vi "Init Any Page.vi"(8 "error in (no error)":errorcluster, 11 "VI in":refnum<vi>) -> (1 "Page Ctrl #N Ref":refnum<vi>, 2 "Page Ctrl #1 Ref":refnum<vi>)   [LabVIEW 2016]
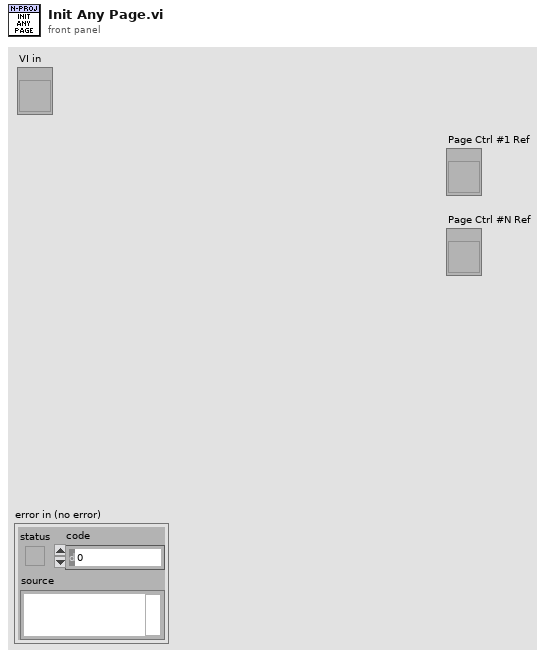
[diagram p1: front panel]
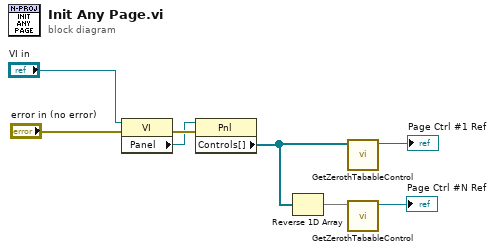
[diagram p0: block diagram]
diagram:
  n1 = property class="VI"(reference="VI in", error in="error in (no error)") -> (error out=w4:errorcluster, "Panel"=w3:refnum<vi>)  [unwired: 1 out]
  n2 = property class="Pnl"(reference=w3, error in=w4) -> ("Controls[]"=w6:refnum<vi>[])  [unwired: 2 out]
  n3 = Reverse 1D Array(array=w6) -> (reversed array=w7:refnum<vi>[])
  n4 = call <resource>:"GetZerothTabableControl.vi"("Controls[]"=w6) -> ("Control out"=→"Page Ctrl #1 Ref":refnum<vi>)  [unwired: 10 in]
  n5 = call <resource>:"GetZerothTabableControl.vi"("Controls[]"=w7) -> ("Control out"=→"Page Ctrl #N Ref":refnum<vi>)  [unwired: 10 in]
